vi "updateMission.vi"(8 "error in (no error)":errorcluster, 11 "PassBuoys in":refnum<class "PassBuoys.lvclass">) -> (0 "error out":errorcluster, 3 "PassBuoys out":refnum<class "PassBuoys.lvclass">)   [LabVIEW 2011, in "PassBuoys.lvclass"]
doc: "Just a filler VI. Other missions have waypoints that change as time goes on, or wind changes, but this one does not. No updating needed."
uses:
  PassBuoys.lvclass
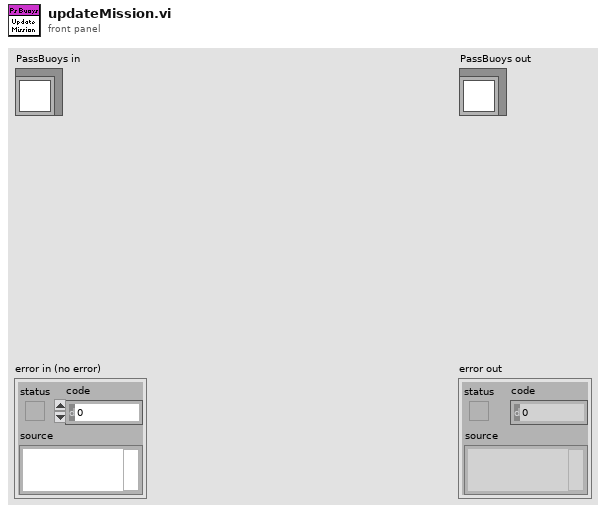
[diagram p1: front panel]
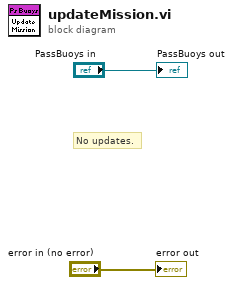
[diagram p0: block diagram]
diagram:
  # "No updates."
  "error out" <- "error in (no error)"
  "PassBuoys out" <- "PassBuoys in"
